vi "PXI-Enumerate DIO Lines (by port).vi"(0 "Direction":enum16{"Input", "Output"}(ring), 7 "Port":string, 9 "change detect":bool, 11 "error in (no error)":errorcluster) -> (4 "Lines":string[](array[string]), 8 "Dev/Port/Lines":tag[](array[tag]), 15 "error out":errorcluster)   [LabVIEW 2020]
uses:
  <resource>/objmgr/daqmx.rc
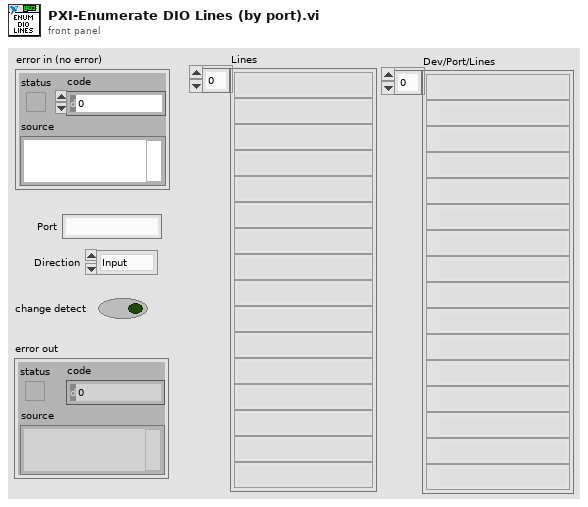
[diagram p1: front panel]
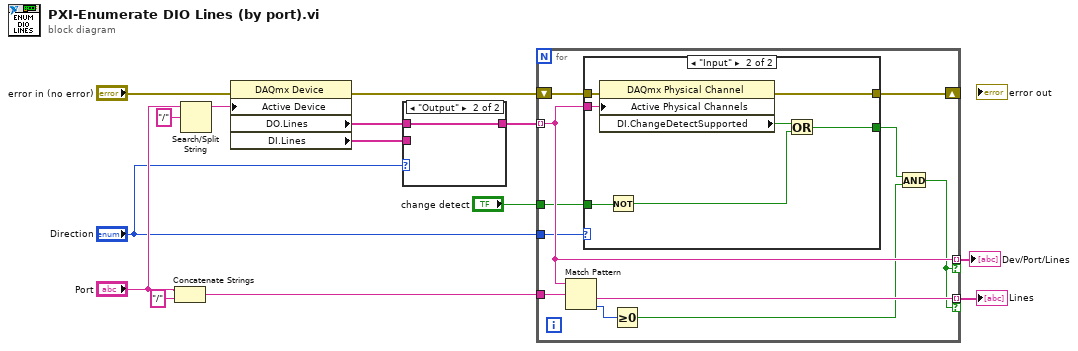
[diagram p0: block diagram]
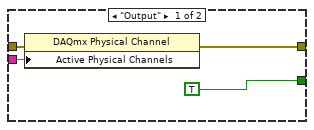
[diagram p2: hidden frame]
diagram:
  n1 = Concatenate Strings("Port", "/" ("string")) -> (w8:string)
  n2 = Search/Split String(string="Port", search string/char (-)="/") -> (substring before match=w12:string)  [unwired: 1 in, 2 out]
  n3 = property class="DAQmx Device"(error in="error in (no error)", "Active Device"=w12) -> (error out=w3:errorcluster, "DO.Lines"=w14:tag[], "DI.Lines"=w6:tag[])  [unwired: 1 in, 1 out]
  n4 = case shown="\"Output\"" "Direction" {
    tunnel: w14 -> [_ w16]
    tunnel: w6 -> [w15 _]
    tunnel: [w15 w16] -> w4
    frame "Input", Default {
    }
    frame "Output" {
    }
  }
  n5 = for {
    tunnel: w4 -> [w22] mode=indexing
    tunnel: w8 -> [w27]
    tunnel: [w26] -> w7 mode=indexing if=w18
    tunnel: [w22] -> w5 mode=indexing if=w18
    shift-right: [w23] -> _
    shift-left: w3 -> [w24]
    tunnel: "Direction" -> [w21]
    tunnel: "change detect" -> [w17]
    n6 = Match Pattern(string=w22, regular expression=w27) -> (after substring=w26:string, offset past match=w25:i32)  [unwired: 1 in, 2 out]
    n7 = case shown="\"Input\"" w21 {
      tunnel: w24 -> [w31 w38]
      tunnel: [w30 w37] -> w23
      tunnel: w22 -> [w29 w36]
      tunnel: [TRUE ("DI.ChangeDetectSupported") w34] -> w20
      tunnel: w17 -> [_ w33]
      frame "Output" {
        n8 = property class="DAQmx Physical Channel"(error in=w31, "Active Physical Channels"=w29) -> (error out=w30:errorcluster)  [unwired: 1 in, 1 out]
      }
      frame "Input" {
        n9 = property class="DAQmx Physical Channel"(error in=w38, "Active Physical Channels"=w36) -> (error out=w37:errorcluster, "DI.ChangeDetectSupported"=w35:bool)  [unwired: 1 in, 1 out]
        n10 = Not(x=w33) -> (.not. x?=w32:bool)
        n11 = Or(x=w35, y=w32) -> (x .or. y?=w34:bool)
      }
    }
    n12 = Greater Or Equal To 0?(x=w25) -> (x >= 0?=w19:bool)
    n13 = And(x=w20, y=w19) -> (x .and. y?=w18:bool)
  }
  "Lines" <- w7
  "Dev/Port/Lines" <- w5
